vi "python_test.vi"() -> ()   [LabVIEW 2018, in "monoDrive.lvlib"]
uses:
  monoDrive.lvlib
panel:
  out "Array":i32[](array[numeric])
  out "Numeric":sgl
  out "String":string
  out "return value":cluster{string, i32, i32[]}
  out "array1 2":sgl
  in  "size_of_array_in 2":sgl
  out "error out":errorcluster
  in  "size_of_array_in":sgl
  in  "array1":sgl[](array[numeric])
  in  "module path":path
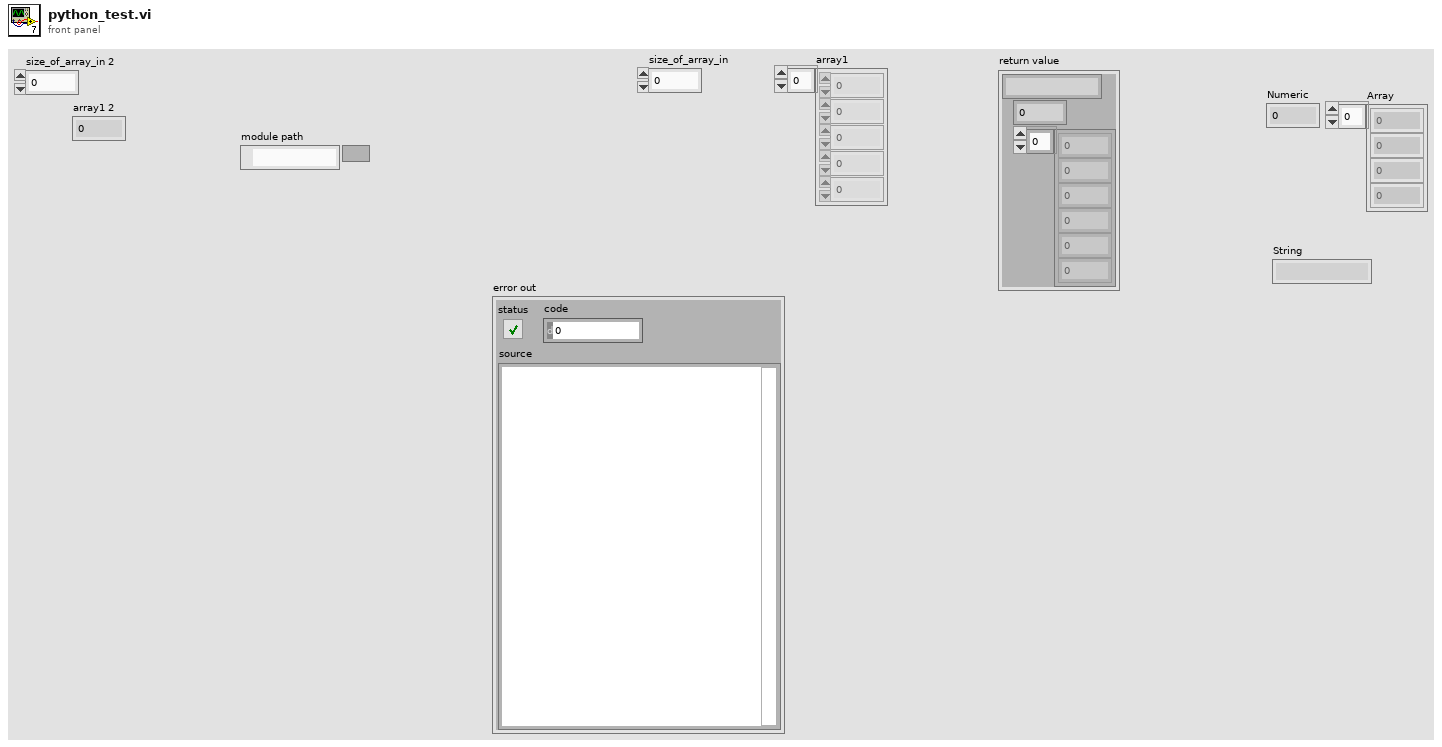
[diagram p1: front panel]
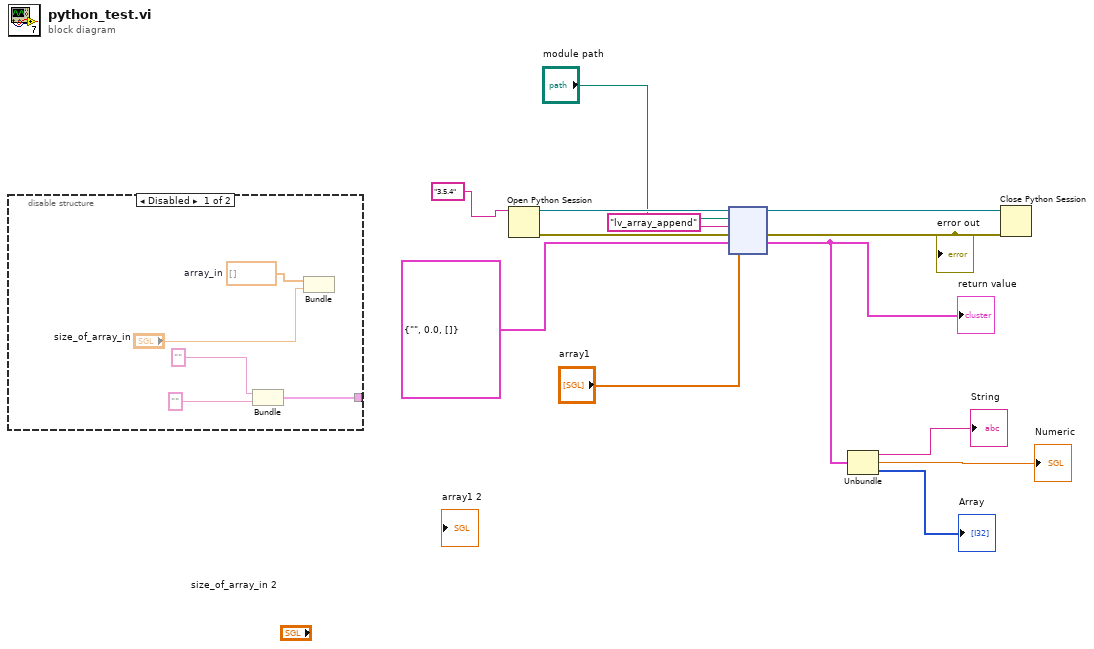
[diagram p0: block diagram]
diagram:
  n1 = disable-structure shown="Disabled" {
    disable-tunnel: [w14 _] -> _
    frame Disabled {
      w18 = sgl[] []  # array_in
      n2 = Bundle("", "") -> (w14:cluster{string, string})  [unwired: 1 in]
      n3 = Bundle("array_in"=w18, "size_of_array_in"="size_of_array_in") -> ()  [unwired: 1 in, 1 out]
    }
    frame Enabled {
    }
  }
  n4 = Open Python Session(python version="3.5.4" ("Python version")) -> (session out=w11:refnum<k35>, error out=w12:errorcluster)  [unwired: 2 in]
  n5 = node(w11, "module path", "lv_array_append" ("function name"), w12, cluster{string, sgl, i32[]} {"", 0.0, []}, "array1") -> (w9:refnum<k35>, w8:errorcluster, w4:cluster{string, sgl, i32[]})  [unwired: 1 in, 2 out]
  "error out" <- w8
  "return value" <- w4
  n6 = Unbundle(w4) -> (→"String":string, →"Numeric":sgl, →"Array":i32[])
  n7 = Close Python Session(session in=w9, error in=w8) -> ()  [unwired: 1 out]
